vi "SVA 4MV6 T012 CCE.vi"() -> ()   [LabVIEW 2020]
panel:
  out "2D Picture 2":picture
  in  "Boolean array":bool[](array[boolean])
  out "R":u8
  out "Color Box":u32(colorbox)
  out "2D Picture":picture
  in  "Path":path
  # "Ceballos Conde Emanuel"
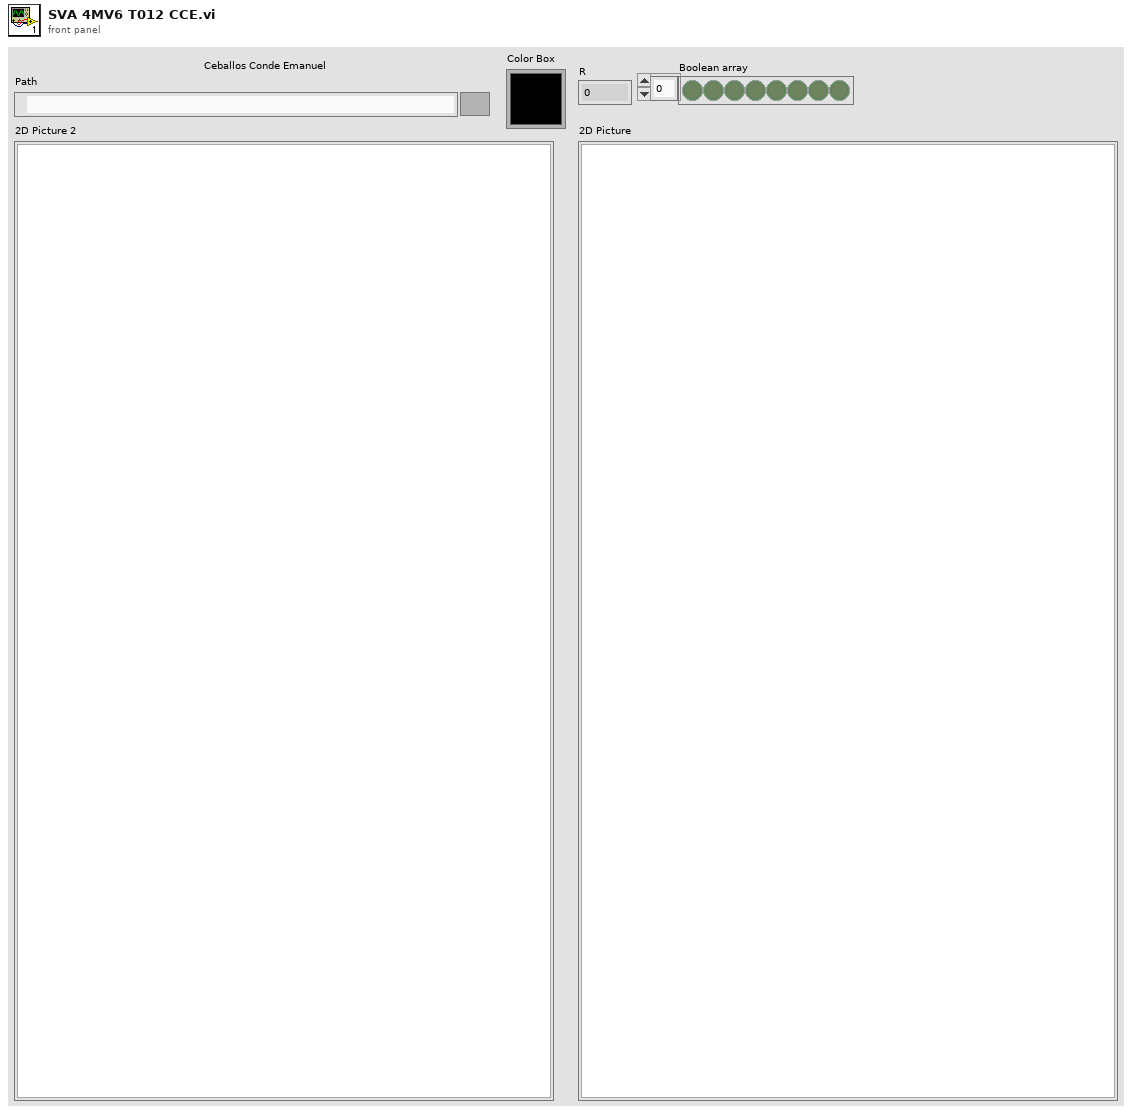
[diagram p1: front panel]
types:
  T1 = typedef "imagedata.ctl" = cluster{"image type":i32, "image depth":i32, "image":u8[], "mask":u8[], "colors":u32[], "Rectangle":cluster{"left":i16, "top":i16, "right":i16, "bottom":i16}}
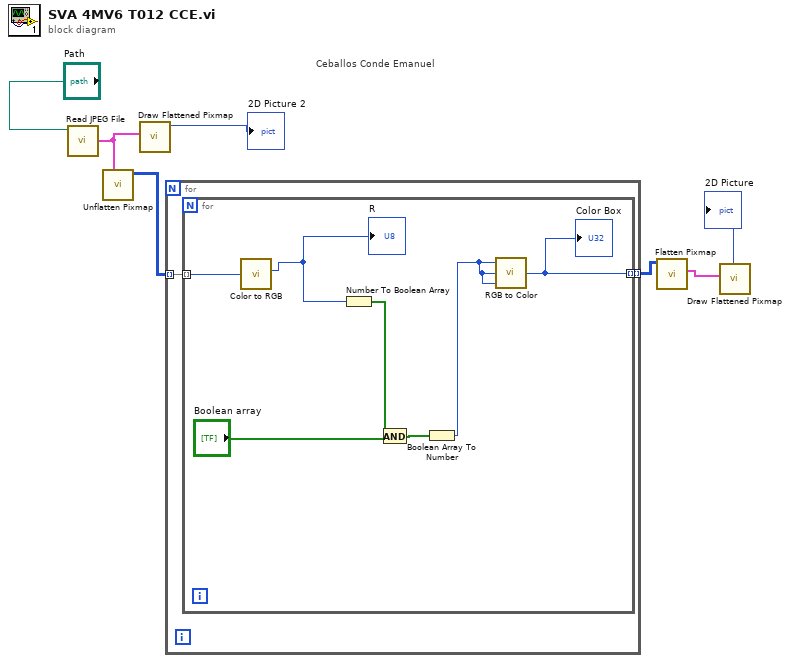
[diagram p0: block diagram]
diagram:
  # "Ceballos Conde Emanuel"
  n1 = call <vilib>:"Read JPEG File.vi"("path to JPEG file"="Path") -> ("image data"=w6:T1)  [unwired: 8 in, 2 out]
  n2 = call <vilib>:"Unflatten Pixmap.vi"("image data"=w6) -> ("24-bit pixmap"=w5:u32[][])  [unwired: 4 in, 6 out]
  n3 = call <vilib>:"Draw Flattened Pixmap.vi"("image data"=w6) -> ("new picture"=→"2D Picture 2":picture)  [unwired: 8 in]
  n4 = for {
    tunnel: w5 -> [w9] mode=indexing
    tunnel: [w8] -> w4 mode=indexing
    n5 = for {
      tunnel: w9 -> [w16] mode=indexing
      tunnel: [w15] -> w8 mode=indexing
      n6 = call <vilib>:"Color to RGB.vi"("Color"=w16) -> ("R"=w11:u8)  [unwired: 3 out]
      "R" <- w11
      n7 = Number To Boolean Array(number=w11) -> (Boolean array=w13:bool[])
      n8 = And(x=w13, y="Boolean array") -> (x .and. y?=w12:bool[])
      n9 = Boolean Array To Number(Boolean array=w12) -> (number=w10:u32)
      n10 = call <vilib>:"RGB to Color.vi"("B"=w10, "G"=w10, "R"=w10) -> ("Color"=w15:u32)
      "Color Box" <- w15
    }
  }
  n11 = call <vilib>:"Flatten Pixmap.vi"("24-bit pixmap"=w4) -> ("image data"=w3:T1)  [unwired: 10 in]
  n12 = call <vilib>:"Draw Flattened Pixmap.vi"("image data"=w3) -> ("new picture"=→"2D Picture":picture)  [unwired: 8 in]
